vi "Encode packed enum.vi"(7 "Field Number":i32, 10 "Enumeration":T1[](array[typedef]), 11 "Buffer in":u8[](array[numeric]) format="%.0x") -> (3 "Buffer":u8[](array[numeric]) format="%.0x")   [LabVIEW 2020, in "ConnectStatus.lvlib"]
uses:
  ConnectStatus.lvlib
  Enumeration.ctl
  lv-protoc/LV-Proto/Wire Type.ctl
  lv-protoc/LV-Proto/LV-Proto.lvlib
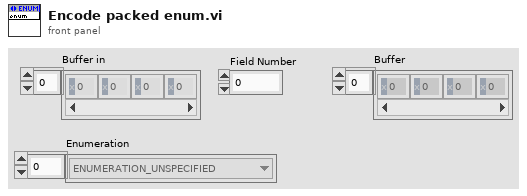
[diagram p1: front panel]
types:
  T1 = typedef "ConnectStatus.lvlib/Enumeration.ctl" = enum16{"ENUMERATION_UNSPECIFIED"}
  T2 = typedef "LV-Proto.lvlib/Wire Type.ctl" = enum8{"VARINT", "I64", "LEN", "SGROUP (Deprecated)", "EGROUP (Deprecated)", "I32"}
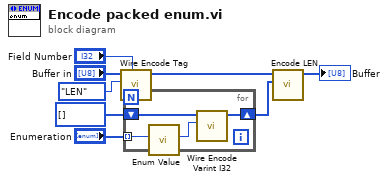
[diagram p0: block diagram]
diagram:
  n1 = call "Wire Encode Tag.vi"("Field Number"="Field Number", "Wire Type"=Wire_Type."LEN", "Buffer in"="Buffer in") -> ("Buffer"=w6:u8[])  [unwired: 8 in]
  n2 = for {
    shift-right: [w10] -> w5
    shift-left: u8[] [] ("Buffer") -> [w12]
    tunnel: "Enumeration" -> [w11] mode=indexing
    n3 = call "Enum Value.vi"("Enumeration"=w11) -> ("Value"=w9:i32)  [unwired: 10 in]
    n4 = call "Wire Encode Varint I32.vi"("I32"=w9, "Buffer in"=w12) -> ("Buffer"=w10:u8[])  [unwired: 9 in]
  }
  n5 = call "Encode LEN.vi"("Data"=w5, "Buffer in"=w6) -> ("Buffer"=→"Buffer":u8[])  [unwired: 9 in]
